vi "ESP Init Pop-up.vi"(8 "Error In":errorcluster, 11 "Address / Port in":i16) -> (0 "Error Out":errorcluster)   [LabVIEW 2014]
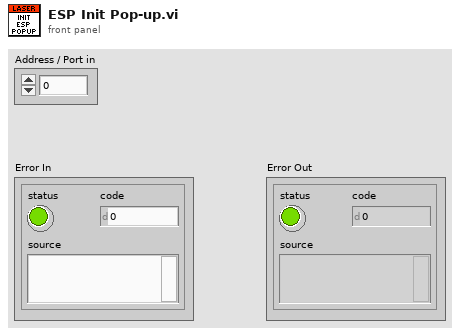
[diagram p1: front panel]
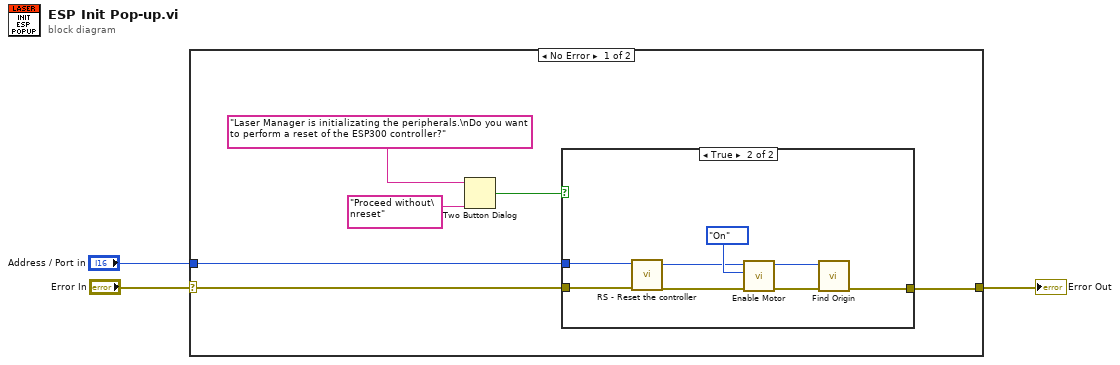
[diagram p0: block diagram]
diagram:
  n1 = case shown="No Error" "Error In" {
    selector: "Error In" -> [w6 w19]
    tunnel: [w5 w19] -> w2
    tunnel: "Address / Port in" -> [w4 _]
    frame No Error {
      n2 = Two Button Dialog(message="Laser Manager is initializating the peripherals.\nDo you want to perform a reset of the ESP300 controller?", 1:"Proceed without\nreset" ("F button name (\"Cancel\")")) -> (T button?=w7:bool)  [unwired: 1 in]
      n3 = case shown="True" w7 {
        tunnel: w6 -> [w10 w13]
        tunnel: [w10 w12] -> w5
        tunnel: w4 -> [_ w11]
        frame False {
        }
        frame True {
          n4 = call "RS - Reset the controller.vi"("error in"=w13, "Address / Port"=w11) -> ("error out"=w16:errorcluster, "Address / Port out"=w17:i16)  [unwired: 6 in]
          n5 = call "Enable Motor.vi"("Error In"=w16, "On/Off"=enum16{"On", "Off"}."On", "Address / Port"=w17) -> ("Error Out"=w15:errorcluster, "Address / Port dup"=w14:i16)  [unwired: 7 in]
          n6 = call "Find Origin.vi"("Error In"=w15, "Address / Port"=w14) -> ("Error Out"=w12:errorcluster)  [unwired: 8 in, 1 out]
        }
      }
    }
    frame Error {
    }
  }
  "Error Out" <- w2
